vi "Data Transform.vi"(9 "dim":i64[](array[numeric])=[1, 5, 21504], 10 "threshold":sgl=0.9, 11 "Array in":sgl[](array[numeric])) -> (3 "Array out":sgl[][](array[numeric]))   [LabVIEW 2017, in "ONNX YOLO Class Library.lvlib"]
doc: "Created IvanLis by LabVIEW Portal\nProfile: http://labviewportal.org/memberlist.php?mode=viewprofile&u=987\neMail: IvanLisanov@gMail.com\nTelegram: https://t.me/IvanLis"
uses:
  ONNX YOLO Class Library.lvlib
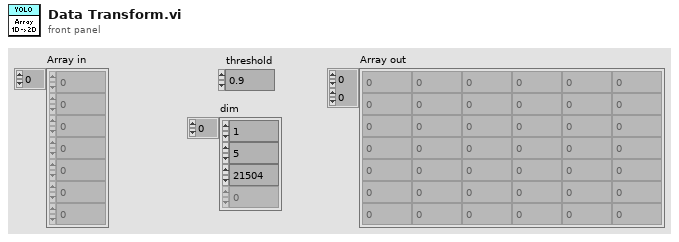
[diagram p1: front panel]
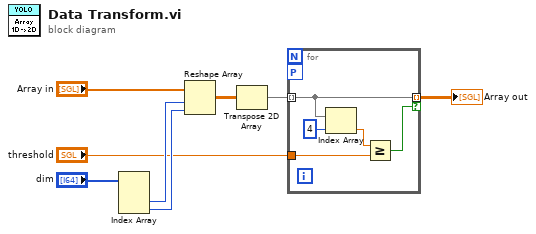
[diagram p0: block diagram]
diagram:
  n1 = Index Array(array="dim") -> (element #2=w7:i64, element #3=w8:i64)  [unwired: 3 in, 1 out]
  n2 = Reshape Array("Array in", w7, w8) -> (w2:sgl[][])
  n3 = Transpose 2D Array(2D array=w2) -> (transposed array=w3:sgl[][])
  n4 = for {
    tunnel: w3 -> [w10] mode=indexing
    tunnel: "threshold" -> [w11]
    workers-P: _ -> [_]
    tunnel: [w10] -> w5 mode=indexing if=w9
    n5 = Index Array(array=w10, index=4) -> (element=w12:sgl)
    n6 = Greater Or Equal?(x=w12, y=w11) -> (x >= y?=w9:bool)
  }
  "Array out" <- w5
